vi "Tracker_v3_test_acq_comms_channel.vi"() -> ()   [LabVIEW 2018]
uses:
  <vilib>/Instr/_visa.llb/Select Event Type.ctl
  <vilib>/Platform/TimedLoop/XDataNode/timing_clust.ctl
  <vilib>/Platform/TimedLoop/XDataNode/nitl_modes.ctl
  <vilib>/Platform/TimedLoop/XDataNode/wakeup.ctl
  <extravilib>/ChannelInstances/High Speed Stream-c(a[.](u16),stamp)/_Read For Replicate.vi
  <vilib>/Platform/TimedLoop/scheduler/LVUserAPI/_suppVIs/Create_1kHz_TSource.vi
  <extravilib>/ChannelInstances/High Speed Stream-c(a[.](u16),stamp)/Instantiate.vi
  <extravilib>/ChannelInstances/High Speed Stream-c(a[.](u16),stamp)/)Channel.vi
  <extravilib>/ChannelInstances/High Speed Stream-c(a[.](u16),stamp)/Abort Signal/Init Signal.vi
  <vilib>/Platform/TimedLoop/XDataNode/XDataNode.xnode
  Tracker.lvlib
  <vilib>/Analysis/NI_AALBase.lvlib
  <vilib>/Platform/TimedLoop/XDataNode/XDNodeRunTimeDep.lvlib
  <extravilib>/ChannelInstances/High Speed Stream-c(a[.](u16),stamp).lvlib
panel:
  out "Data frame channel sink":cluster{u16[], "Timestamp":timestamp} {"?" format="%x"}
  out "Time to process, us":dbl format="%0.2f"
  out "standard deviation":dbl format="%0.3f"
  out "mean frame time, ms":dbl format="%0.3f"
  out "count":i32
  out "Instrument OK?":bool=TRUE
  out "Data frame channel source":T1
  in  "Play/Pause":bool
  in  "Stop Button":bool
  in  "VISA resource name in":refnum<visa-resource-name>="ASRL3::INSTR"
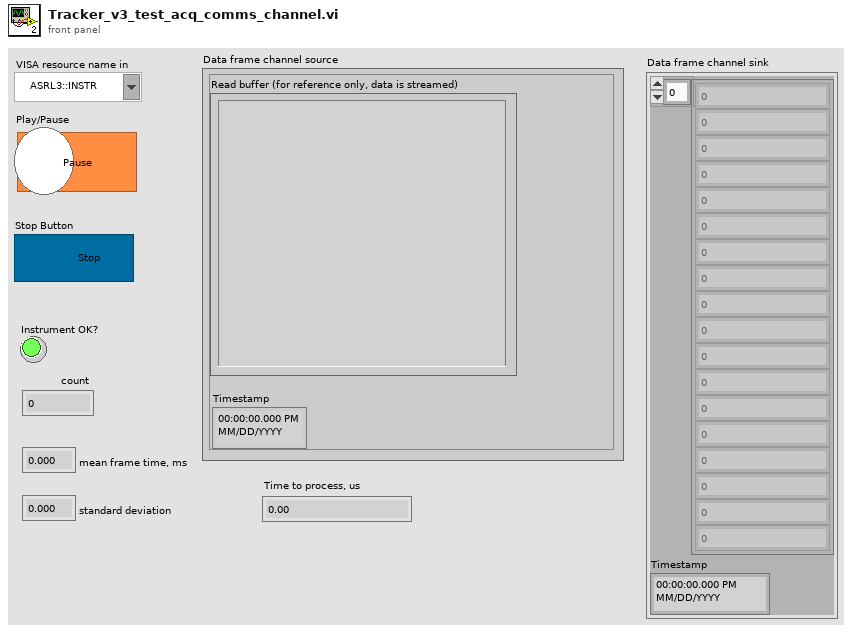
[diagram p1: front panel]
types:
  T1 = cluster{"Read buffer (for reference only, data is streamed)":string, "Timestamp":timestamp}
  T2 = typedef "Select Event Type.ctl" = u32
  T3 = typedef "Common_Resources.lvlib/CTL_Data_flow_control_cluster.ctl" = cluster{"Data acquisition status":refnum<notifier>, "Play/Pause status":refnum<notifier>, "Complete stop":refnum<notifier>, "Temp file ready for processing":refnum<notifier>, "Has been recorded":refnum<notifier>, "Recording now":refnum<notifier>, "Path to the latest complete temp file":refnum<notifier>, "(Final) Data file is saved":refnum<notifier>, "Data loaded":refnum<notifier>}
  T4 = typedef "XDNodeRunTimeDep.lvlib/timing_clust.ctl" = cluster{"Expected End [f-1]":u64, "Actual End [f-1]":u64, "Finished Late? [f-1]":bool, "Expected End [i-1]":u64, "Actual End [i-1]":u64, "Finished Late? [i-1]":bool, "Expected Start [i]":u64, "Actual Start [i]":u64, "Expected Start [f]":u64, "Actual Start [f]":u64, "Source Name":string, "Structure Name":string, "Period":i64, "Deadline":i64, "Offset":i64, "Start":i64, "Priority":i32, "Timeout":i32, "Mode":T5, "Wakeup Reason":T6, "Error":errorcluster, "Source Type":string, "Secondary Source Type":string, "Global End Time":u64, "Global Start Time":u64, "Frame Duration":u64, "Iteration Duration":u64, "Assigned CPU":i32, "I/O Scan Engine Mode":u32}
  T5 = typedef "XDNodeRunTimeDep.lvlib/nitl_modes.ctl" = enum32{"No Change", "Process missed periods, maintain original phase", "Discard missed periods, maintain original phase", "Process missed periods, ignore original phase", "Discard missed periods, ignore original phase"}
  T6 = typedef "XDNodeRunTimeDep.lvlib/wakeup.ctl" = enum32{"Normal", "Aborted", "Asynchronous wakeup", "Timing source error", "Timed loop error", "Timeout"}
  T7 = typedef "High Speed Stream-c(a[.](u16),stamp).lvlib/)Channel.ctl" = refnum<queue>
  T8 = cluster{"Data acquisition status":refnum<notifier>, "Play/Pause status":refnum<notifier>, "Complete stop":refnum<notifier>, "Temp file ready for processing":refnum<notifier>, "Has been recorded":refnum<notifier>, "Recording now":refnum<notifier>, "Path to the latest complete temp file":refnum<notifier>, "Final CSV saved":refnum<notifier>, "Data loaded":refnum<notifier>}
  T9 = cluster{u16[], "seconds since 1Jan1904":timestamp}
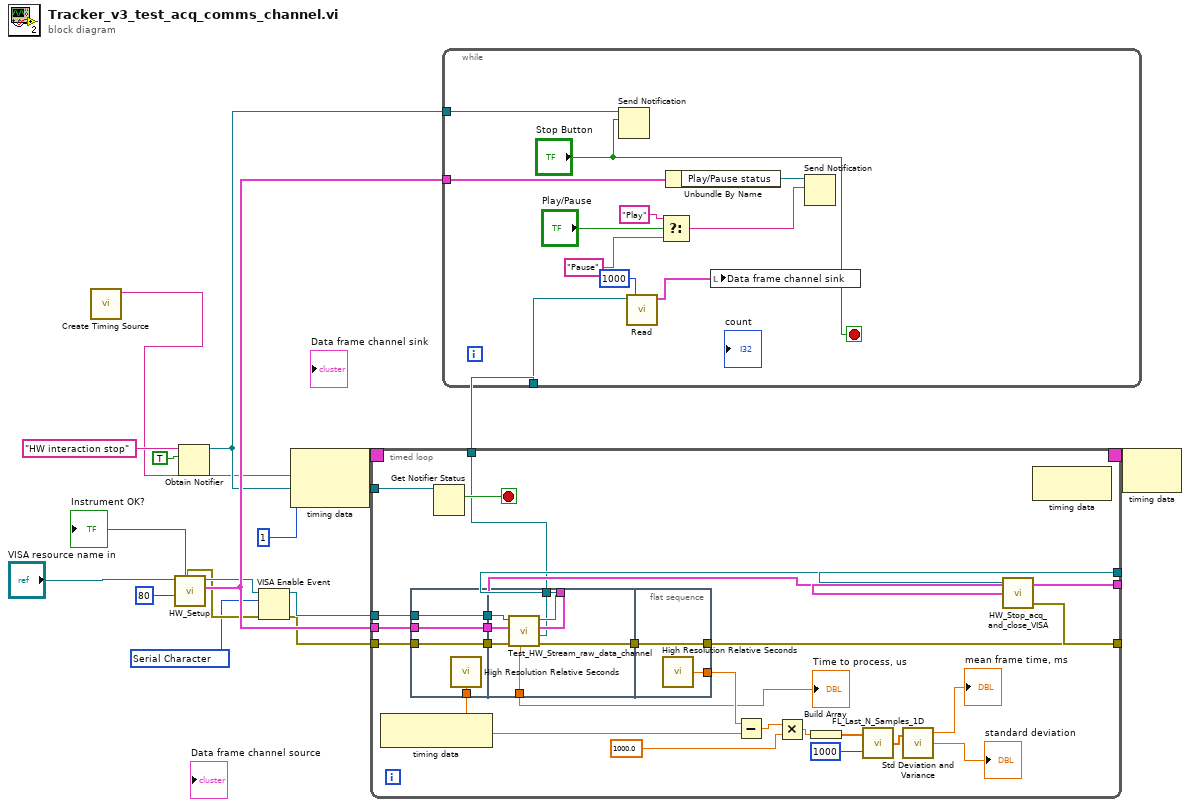
[diagram p0: block diagram]
diagram:
  w3 = T2 1073684533 items=["Service Request"=1073684491, "Trigger"=3221168138, "Clear"=1073684493, "VXI Signal"=1073684512, "VXI/VME Interrupt"=3221168161, "VXI/VME Sysfail"=1073684509, "VXI/VME Sysreset"=1073684510, "GPIB CIC"=1073684498, "GPIB Talk"=1073684499, "GPIB Listen"=1073684500, "PXI Interrupt"=1073684514, "Serial Break"=1073684515, "Serial TermChar"=1073684516, "Serial CTS"=1073684521, "Serial DSR"=1073684522, "Serial DCD"=1073684524, "Serial RI"=1073684526, "Serial Character"=1073684533, "USB Interrupt"=1073684535, "All Enabled"=1073709055] ("Event Type")
  n1 = call-poly <vilib>:"Create Timing Source.vi"() -> ("name (out)"=w10:string)  [unwired: 10 in, 1 out]
  n2 = call "HW_Setup.vi"("Traget FPS"=80, "VISA resource name in"="VISA resource name in") -> ("Instrument OK?"=→"Instrument OK?":bool, "Data flow controls"=w18:T3, "VISA resource name out"=w7:refnum<visa-resource-name>, "error out"=w5:errorcluster)  [unwired: 2 in, 4 out]
  n3 = Obtain Notifier(name (unnamed)="HW interaction stop", notification data type=TRUE) -> (notifier out=w15:refnum<notifier>)  [unwired: 2 in, 2 out]
  n4 = VISA Enable Event(8:w5, 10:w3, 11:w7) -> (0:w4:errorcluster, 3:w6:refnum<visa-resource-name>)  [unwired: 1 in]
  n5 = node-c288(w10, i64 1 ("Period")) -> (w12:T4)
  n6 = timed-loop {
    tunnel: w6 -> [w44]
    tunnel: [w41] -> w1
    tunnel: w18 -> [w43]
    tunnel: [w40] -> w19
    tunnel: w4 -> [w42]
    tunnel: [w37] -> w2
    tunnel: w15 -> [w39]
    tunnel: [w36] -> w14
    timing: w12 -> [_]
    timing-out: [_] -> w11
    stop <- w38 stop-if-true
    n7 = node-c288() -> ()  [unwired: 1 in, 1 out]
    n8 = flat-sequence {
      tunnel: w42 -> [w48]
      tunnel: w43 -> [w49]
      tunnel: w44 -> [w50]
      tunnel: [w50] -> w35
      tunnel: [w49] -> w34
      tunnel: [w48] -> w33
      tunnel: [w47] -> w30
      tunnel: [w55] -> w41
      tunnel: [w54] -> w40
      tunnel: [w52] -> w36
      tunnel: w35 -> [w58]
      tunnel: w34 -> [w57]
      tunnel: w33 -> [w56]
      tunnel: [w53] -> w32
      tunnel: [w51] -> w21
      tunnel: [w60] -> w37
      tunnel: w32 -> [w60]
      tunnel: [w59] -> w31
      frame #0 {
        n9 = call <vilib>:"High Resolution Relative Seconds.vi"() -> ("relative seconds"=w47:dbl)
      }
      frame #1 {
        n10 = call "Test_HW_Stream_raw_data_channel.vi"("error in"=w56, "Data flow controls in"=w57, "VISA resource name in"=w58) -> ("error out"=w53:errorcluster, "High-speed channel"=w52:T7, "Data flow controls out"=w54:T8, "VISA resource name out"=w55:refnum<visa-resource-name>, "Time to process, us"=w51:dbl)  [unwired: 3 in, 1 out]
      }
      frame #2 {
        n11 = call <vilib>:"High Resolution Relative Seconds.vi"() -> ("relative seconds"=w59:dbl)
      }
    }
    n12 = Get Notifier Status(notifier=w39) -> (current notification=w38:bool)  [unwired: 1 in, 4 out]
    n13 = Subtract(x=w31, y=w30) -> (x-y=w29:dbl)
    n14 = Multiply(x=w29, y=1000.0) -> (x*y=w22:dbl)
    n15 = Build Array(w22) -> (w27:dbl[])
    n16 = call "FL_Last_N_Samples_1D.vi"("BufferLengthSamples"=u32 1000, "Input Array"=w27) -> ("Output Array"=w26:dbl[])
    n17 = call <vilib>:"Std Deviation and Variance.vi"("X"=w26) -> ("mean"=→"mean frame time, ms":dbl, "standard deviation"=→"standard deviation":dbl)  [unwired: 1 in, 1 out]
    n18 = node-c288() -> ()  [unwired: 1 in, 1 out]
    "Time to process, us" <- w21
  }
  n19 = while {
    tunnel: w18 -> [w71]
    tunnel: w15 -> [w65]
    tunnel: w14 -> [w63]
    stop <- "Stop Button" stop-if-true
    n20 = Send Notification(notification="Stop Button", notifier=w65) -> ()  [unwired: 1 in, 2 out]
    n21 = call <extravilib>:"Read.vi"("timeout in ms (-1)"=1000, "channel"=w63) -> ("element"=w61:T9)  [unwired: 5 in, 4 out]
    n22 = Select(t="Play", s="Play/Pause", f="Pause") -> (s? t:f=w68:string)
    n23 = Unbundle By Name(w71) -> ("Play/Pause status"=w70:refnum<notifier>)
    n24 = local write "Data frame channel sink"(w61) -> ()
    n25 = Send Notification(notification=w68, notifier=w70) -> ()  [unwired: 1 in, 2 out]
  }
  n26 = call "HW_Stop_acq_and_close_VISA.vi"("error in"=w2, "Data flow controls in"=w19, "VISA resource name in"=w1) -> ()  [unwired: 2 out]
  n27 = node-c288(w11) -> ()  [unwired: 1 out]
